vi "RaiseIndex.vi"(8 "error in (no error)":errorcluster, 10 "x":i64, 11 "MsgPackDeserializer in":refnum<class "MsgPackDeserializer.lvclass">) -> (0 "error out":errorcluster, 3 "MsgPackDeserializer out":refnum<class "MsgPackDeserializer.lvclass">)   [LabVIEW 2015, in "MsgPackDeserializer.lvclass"]
uses:
  MsgPackDeserializer.lvclass
  MsgPackDeserializer.lvclass/MsgPackDeserializer.ctl
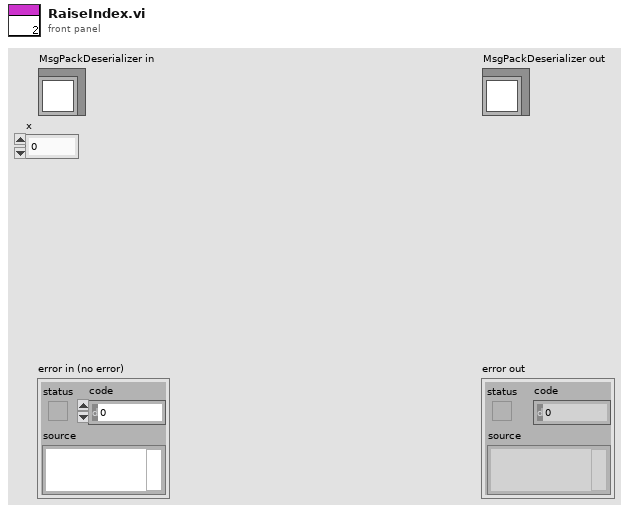
[diagram p1: front panel]
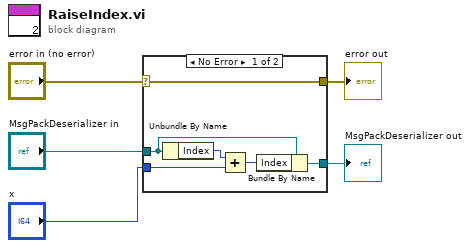
[diagram p0: block diagram]
diagram:
  n1 = case shown="No Error" "error in (no error)" {
    selector: "error in (no error)" -> [w11 w13]
    tunnel: [w11 w13] -> w4
    tunnel: [w6 w12] -> w2
    tunnel: "MsgPackDeserializer in" -> [w10 w12]
    tunnel: "x" -> [w7 _]
    frame No Error {
      n2 = Unbundle By Name(w10) -> ("Index"=w9:i64)
      n3 = Add(x=w9, y=w7) -> (x+y=w8:i64)
      n4 = Bundle By Name(cluster=w10, "Index"=w8) -> (w6:refnum<class "MsgPackDeserializer.lvclass">)
    }
    frame Error {
    }
  }
  "error out" <- w4
  "MsgPackDeserializer out" <- w2
